vi "Status Temperature Setpoint.vi"(8 "error in (no error)":errorcluster, 11 "heater_explorer in":refnum<class "heater_explorer.lvclass">) -> (0 "error out":errorcluster, 2 "Setpoint":dbl, 3 "heater_explorer out":refnum<class "heater_explorer.lvclass">)   [LabVIEW 2020, in "polar_bear_plus_drivers.lvlib" / "heater_explorer.lvclass"]
doc: "Get the current setpoint."
uses:
  <instrlib>/RxnRover/Driver Polar Bear Plus/heater_explorer/heater_explorer.lvclass
  <instrlib>/RxnRover/Driver Polar Bear Plus/heater_explorer/heater_explorer.lvclass/heater_explorer.ctl
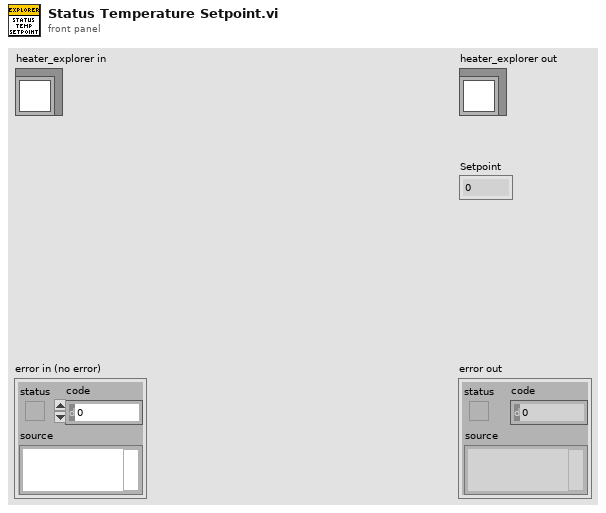
[diagram p1: front panel]
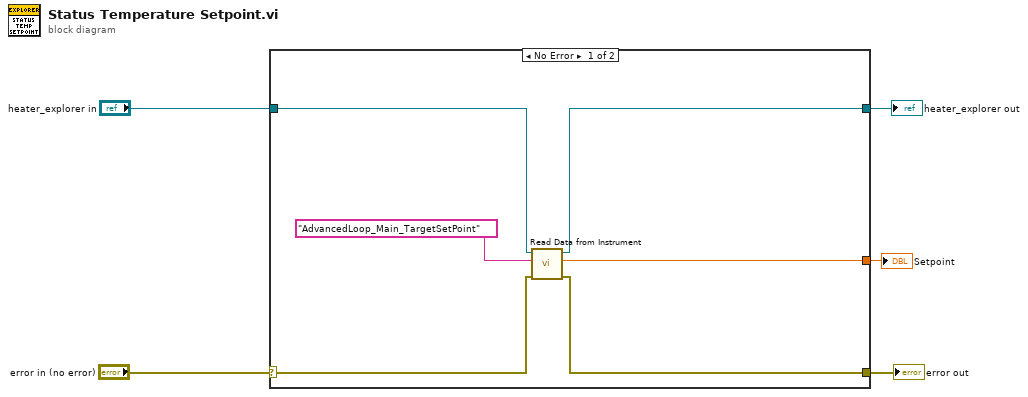
[diagram p0: block diagram]
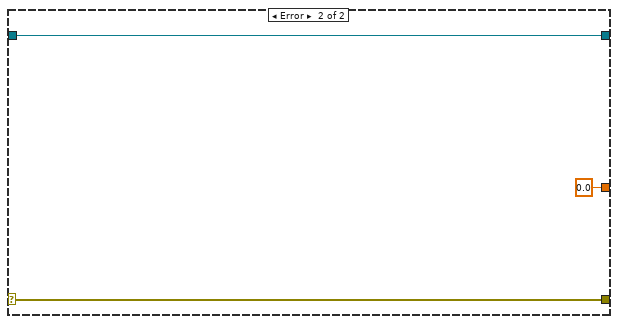
[diagram p2: hidden frame]
diagram:
  n1 = case shown="No Error" "error in (no error)" {
    selector: "error in (no error)" -> [w10 w14]
    tunnel: [w9 w14] -> w5
    tunnel: [w8 w13] -> w3
    tunnel: "heater_explorer in" -> [w11 w13]
    tunnel: [w6 0.0 ("Value Read")] -> w4
    frame No Error {
      n2 = call-dynamic "Read Data from Instrument.vi"("error in (no error)"=w10, "Address"="AdvancedLoop_Main_TargetSetPoint", "heater_parent in"=w11) -> ("error out"=w9:errorcluster, "Value Read"=w6:dbl, "heater_parent out"=w8:refnum<class "heater_explorer.lvclass">)  [unwired: 6 in]
    }
    frame Error {
    }
  }
  "error out" <- w5
  "heater_explorer out" <- w3
  "Setpoint" <- w4
